vi "Control IR Emitter.vi"(0 "Session Handle in":T1, 7 "Start?":bool, 11 "error in (no error)":errorcluster) -> (4 "Session Handle out":T1, 6 "Success?":bool, 8 "Error Code":string, 15 "error out":errorcluster)   [LabVIEW 2015, in "PAS.lvclass"]
uses:
  PAS.lvclass
  Typedefs/Session Handle.ctl
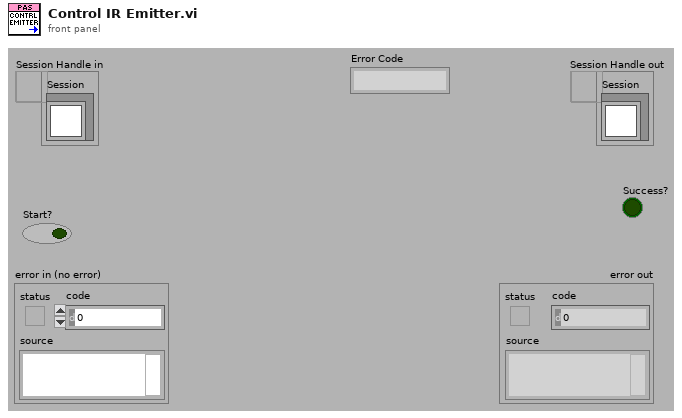
[diagram p1: front panel]
types:
  T1 = typedef "PAS.lvclass/Session Handle.ctl" = refnum<data-value>
  T2 = typedef "XNET Frame CAN.ctl" = cluster{"timestamp":timestamp, "payload":u8[], "identifier":u32, "type":T3, "extended?":bool, "echo?":bool}
  T3 = typedef "XNET Frame Type CAN.ctl" = u8
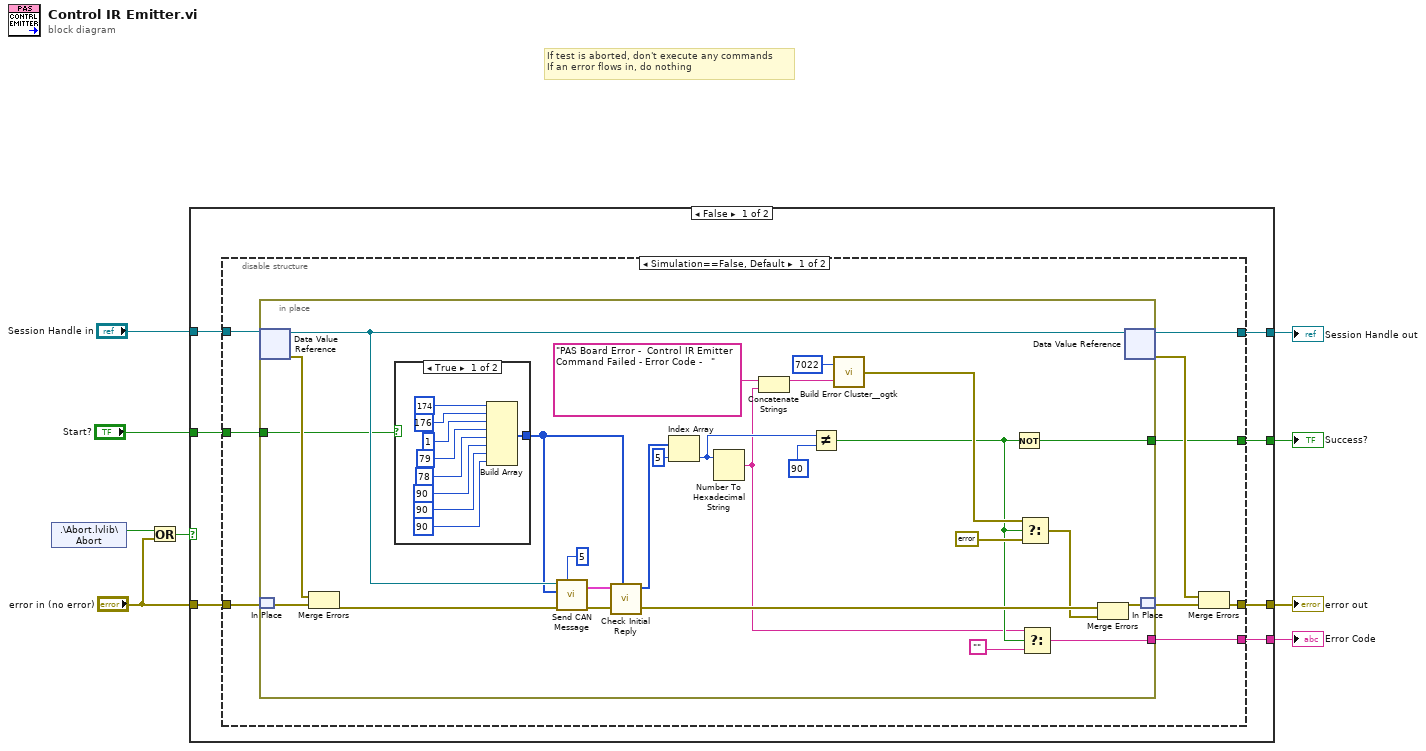
[diagram p0: block diagram]
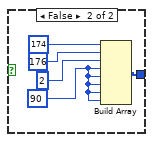
[diagram p2: hidden frame]
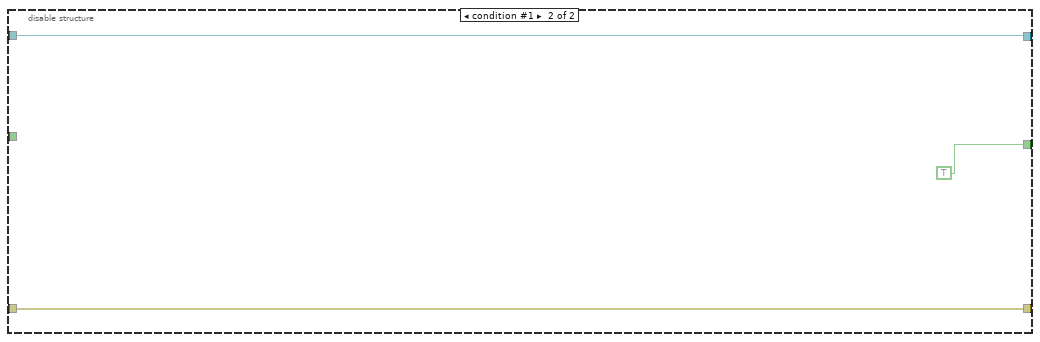
[diagram p3: hidden frame]
diagram:
  # "If test is aborted, don't execute any commands\nIf an error flows in, do nothing"
  n1 = shared-variable ".\\Abort.lvlib\\Abort"() -> (w6:bool)  [unwired: 1 in, 1 out]
  n2 = Or(x=w6, y="error in (no error)") -> (x .or. y?=w4:bool)
  n3 = case shown="False" w4 {
    tunnel: [w16 w69] -> w8
    tunnel: [w15 w68] -> w7
    tunnel: "Session Handle in" -> [w14 w69]
    tunnel: "error in (no error)" -> [w13 w68]
    tunnel: [w12 _] -> w3
    tunnel: "Start?" -> [w11 _]
    tunnel: [w10 _] -> w1
    frame False {
      n4 = disable-structure shown="Simulation==False, Default" {
        disable-tunnel: [w25 w67] -> w16
        disable-tunnel: [w22 w66] -> w15
        disable-tunnel: w14 -> [w21 w67]
        disable-tunnel: w13 -> [w20 w66]
        disable-tunnel: [w19 TRUE] -> w12
        disable-tunnel: w11 -> [w18 _]
        disable-tunnel: [w17 _] -> w10
        frame condition #0 (active) {
          n5 = in-place {
            in-place-border: [w40] -> w19
            in-place-border: w18 -> [w39]
            in-place-border: [w26] -> w17
            n6 = in-place-dvr #1(w21) -> (w46:refnum<class "PAS.lvclass">, w49:errorcluster)
            n7 = in-place-match #2(w20) -> (w48:errorcluster)
            n8 = Merge Errors(w49, w48) -> (w47:errorcluster)
            n9 = case shown="True" w39 {
              tunnel: [w55 w62] -> w38
              frame True {
                n10 = Build Array(u8 174 ("new element/subarray"), u8 176 ("new element/subarray"), u8 1 ("new element/subarray"), u8 79 ("new element/subarray"), u8 78 ("new element/subarray"), u8 90 ("new element/subarray"), u8 90 ("new element/subarray"), u8 90 ("new element/subarray")) -> (w55:u8[])
              }
              frame False {
                w60 = u8 90 ("new element/subarray")
                n11 = Build Array(u8 174 ("new element/subarray"), u8 176 ("new element/subarray"), u8 2 ("new element/subarray"), w60, w60, w60, w60, w60) -> (w62:u8[])
              }
            }
            n12 = call "Send CAN Message.vi"("Number of Retries"=5, "error in (no error)"=w47, "payload"=w38, "Gas In"=w46) -> ("error out"=w31:errorcluster, "Reply"=w44:T2[])  [unwired: 5 in, 1 out]
            n13 = call "Check Initial Reply.vi"("Write Message"=w38, "Reply"=w44) -> ("Data Packet"=w37:u8[])  [unwired: 7 in, 2 out]
            n14 = Index Array(array=w37, index=5) -> (element=w33:u8)
            n15 = Number To Hexadecimal String(2:w33) -> (0:w27:string)  [unwired: 1 in]
            n16 = Concatenate Strings("PAS Board Error -  Control IR Emitter Command Failed - Error Code -   " ("string"), w27) -> (w34:string)
            n17 = Not Equal?(x=w33, y=u8 90 ("new element/subarray")) -> (x != y?=w28:bool)
            n18 = call <userlib>:"Build Error Cluster__ogtk.vi"("String to Prepend to source (\"\")"=w34, "code"=7022) -> ("error out"=w42:errorcluster)
            n19 = Not(x=w28) -> (.not. x?=w40:bool)
            n20 = Select(t=w42, s=w28, f=errorcluster {"status"=FALSE, "code"=0, "source"=""}) -> (s? t:f=w30:errorcluster)
            n21 = Select(t=w27, s=w28, f="") -> (s? t:f=w26:string)
            n22 = Merge Errors(w31, w30) -> (w50:errorcluster)
            n23 = in-place-dvr #1(w46) -> (w25:T1, w23:errorcluster)
            n24 = in-place-match #2(w50) -> (w24:errorcluster)
          }
          n25 = Merge Errors(w23, w24) -> (w22:errorcluster)
        }
        frame condition #1 {
        }
      }
    }
    frame True {
    }
  }
  "Session Handle out" <- w8
  "error out" <- w7
  "Success?" <- w3
  "Error Code" <- w1
